vi "Build Path - Write.vi"(1 "Directory":path) -> (0 "Path to Write.vi":path)   [LabVIEW 2020]
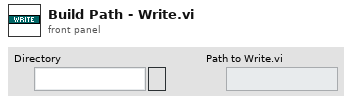
[diagram p1: front panel]
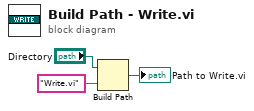
[diagram p0: block diagram]
diagram:
  n1 = Build Path(base path="Directory", name or relative path="Write.vi" ("Selector Name")) -> (appended path=→"Path to Write.vi":path)
